vi "GetErrorDescription.vi"(8 "error in (no error)":errorcluster, 11 "Value":string) -> (0 "error out":errorcluster, 2 "description":string, 3 "Found":bool)   [LabVIEW 2021]
uses:
  87a86f07-fc27-49c6-b2de-2965638c379d.vi
  <vilib>/JDP Science/JSONtext/Find Item.vi
  <vilib>/JDP Science/JSONtext/Next JSON Value.vi
  <vilib>/JDP Science/JSONtext/String Subset.vi
  <vilib>/JDP Science/JSONtext/Parsing/Advance past next JSON Value (inlined COPY).vi
  <vilib>/JDP Science/JSONtext/Parsing/Advance past whitespace.vi
  <vilib>/JDP Science/JSONtext/Parsing/Advance past String.vi
  <vilib>/JDP Science/JSONtext/Parsing/Advance past Number.vi
  <vilib>/JDP Science/JSONtext/Parsing/Advance past Line Ending.vi
  <vilib>/JDP Science/JSONtext/Parsing/Parse Full Path or Item Name.vi
  <vilib>/JDP Science/JSONtext/Parsing/Advance past Array.vi
  <vilib>/JDP Science/JSONtext/Parsing/Advance past Object.vi
  <vilib>/JDP Science/JSONtext/support/Error Cluster From Code.vi
  <vilib>/JDP Science/JSONtext/Offset/Find Item Locations by Path.vi
  <vilib>/JDP Science/JSONtext/JSON text to Variant.vi
  <vilib>/JDP Science/JSONtext/LVClass Serializer/JSONtext LVClass Serializer.lvclass
panel:
  out "decimal integer string":string
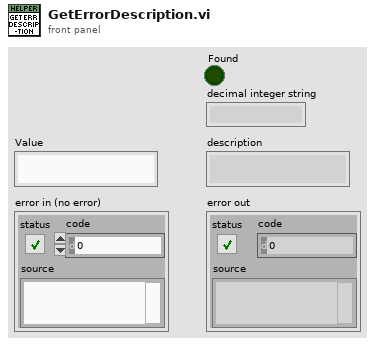
[diagram p1: front panel]
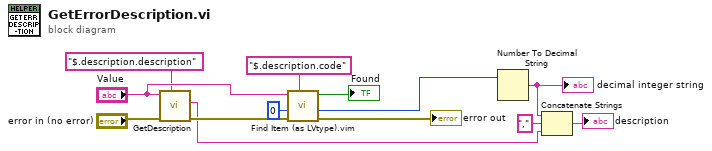
[diagram p0: block diagram]
diagram:
  n1 = call "GetDescription.vi"("$Path or Item Name"="$.description.description", "error in (no error)"="error in (no error)", "Value"="Value") -> ("error out"=w3:errorcluster, "description"=w2:string)  [unwired: 7 in]
  n2 = call "Find Item (as LVtype).vim"("$Path or Item Name"="$.description.code", "error in (no error)"=w3, "Data Type and Default Value"=0, "JSON"="Value") -> ("error out"=→"error out":errorcluster, "Data"=w10:i32, "Found"=→"Found":bool)  [unwired: 4 in, 1 out]
  n3 = Number To Decimal String(number=w10) -> (decimal integer string=w9:string)  [unwired: 1 in]
  "decimal integer string" <- w9
  n4 = Concatenate Strings(w9, "," ("string"), w2) -> (→"description":string)
